vi "Register Events to Controller.vi"(8 "error in (no error)":errorcluster, 11 "View Actor in":refnum<class "View Actor.lvclass">) -> (0 "error out":errorcluster, 3 "View Actor out":refnum<class "View Actor.lvclass">)   [LabVIEW 2017, in "Event Actors.lvlib" / "View Actor.lvclass"]
doc: "This dynamic dispatch method has to be overridden by the child View classes to register events to the Controller."
uses:
  View Actor.lvclass
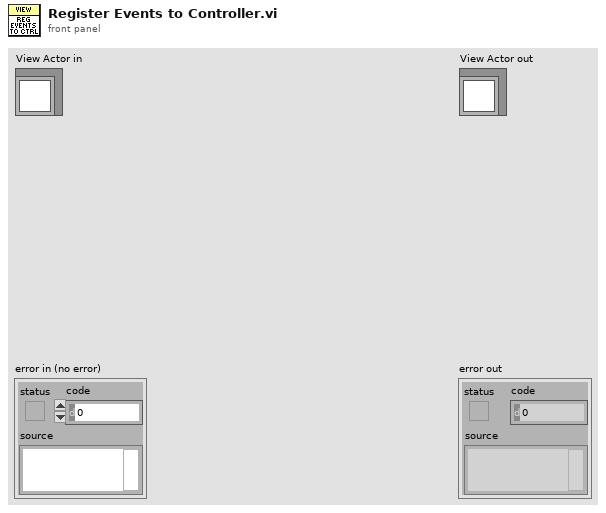
[diagram p1: front panel]
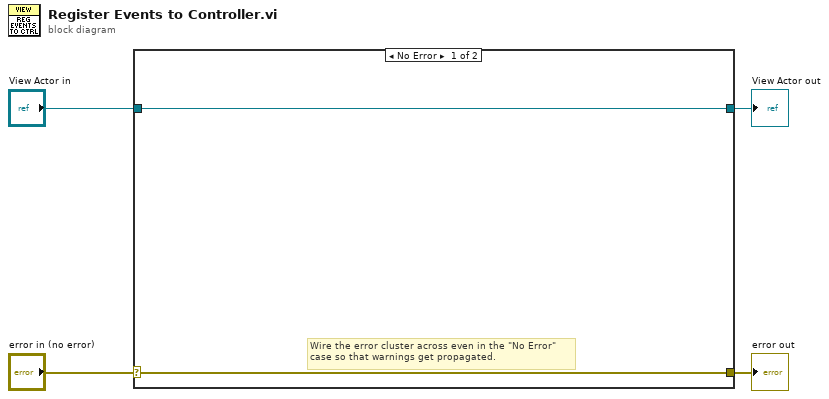
[diagram p0: block diagram]
diagram:
  n1 = case shown="No Error" "error in (no error)" {
    selector: "error in (no error)" -> [w5 w8]
    tunnel: [w5 w8] -> w3
    tunnel: [w6 w7] -> w1
    tunnel: "View Actor in" -> [w6 w7]
    frame No Error {
      # "Wire the error cluster across even in the \"No Error\"\ncase so that warnings get propagated."
    }
    frame Error {
    }
  }
  "error out" <- w3
  "View Actor out" <- w1
